vi "doAction.vi"(8 "error in (no error)":errorcluster, 10 "ContextData":refnum<class "ContextData.lvclass">, 11 "Exit in":refnum<class "Exit.lvclass">) -> (0 "error out":errorcluster, 2 "ContextData Out":refnum<class "ContextData.lvclass">, 3 "Exit out":refnum<class "Exit.lvclass">)   [LabVIEW 2019, in "Exit.lvclass"]
uses:
  Exit.lvclass
  ContextData/ContextData.lvclass
  State/State.lvclass
  Messages/simonMessages/simonMessages.lvclass
  Simon_Engine/Simon_Engine.lvclass
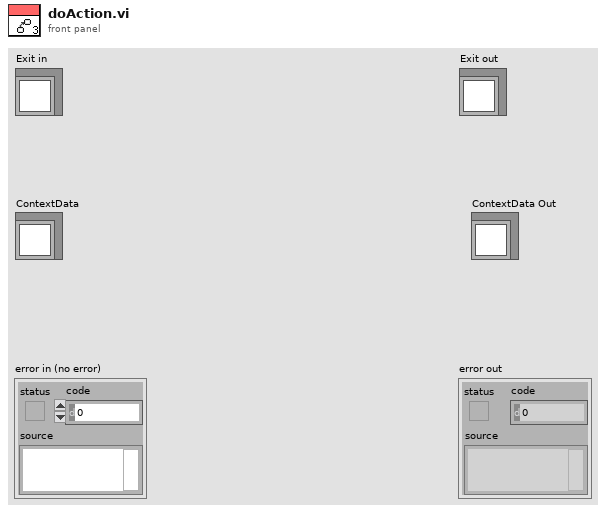
[diagram p1: front panel]
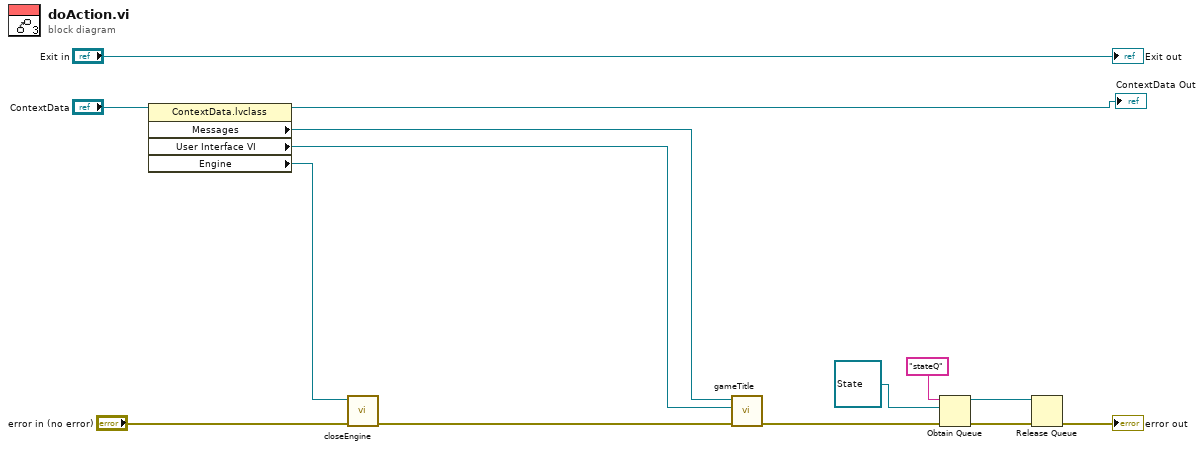
[diagram p0: block diagram]
diagram:
  n1 = property class="ContextData.lvclass"(reference="ContextData") -> (reference out=→"ContextData Out":refnum<class "ContextData.lvclass">, "Messages"=w1:refnum<class "simonMessages.lvclass">, "User Interface VI"=w2:refnum<vi>, "Engine"=w5:refnum<class "Simon_Engine.lvclass">)  [unwired: 1 in, 1 out]
  n2 = call-dynamic "closeEngine.vi"("error in (no error)"="error in (no error)", "Simon_Engine in"=w5) -> ("error out"=w8:errorcluster)  [unwired: 8 in, 1 out]
  n3 = call "gameTitle.vi"("error in (no error)"=w8, "VI Refnum"=w2, "simonMessages in"=w1) -> ("error out"=w6:errorcluster)  [unwired: 7 in, 1 out]
  n4 = Obtain Queue(name (unnamed)="stateQ", element data type=refnum<class "State.lvclass"> refnum ("State.lvclass"), error in (no error)=w6) -> (queue out=w9:refnum<queue>, error out=w13:errorcluster)  [unwired: 2 in, 1 out]
  n5 = Release Queue(queue=w9, error in (no error)=w13) -> (error out=→"error out":errorcluster)  [unwired: 1 in, 2 out]
  "Exit out" <- "Exit in"
